vi "Read OPC UA Client Refnum.vi"(8 "error in (no error)":errorcluster, 11 "UA Server in":refnum<class "UA Server.lvclass">) -> (0 "error out":errorcluster, 2 "OPC UA client refnum":T1, 3 "UA Server out":refnum<class "UA Server.lvclass">)   [LabVIEW 2017, in "Browser Core.lvlib" / "UA Server.lvclass"]
uses:
  UA Server.lvclass
  <vilib>/OPCUA/controls/OPC UA Client Refnum.ctl
  UA Server.lvclass/UA Server.ctl
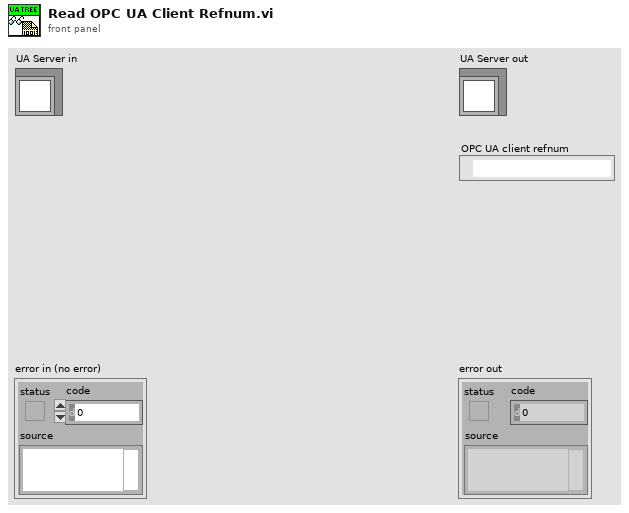
[diagram p1: front panel]
types:
  T1 = typedef "OPC UA Client Refnum.ctl" = refnum<k21>
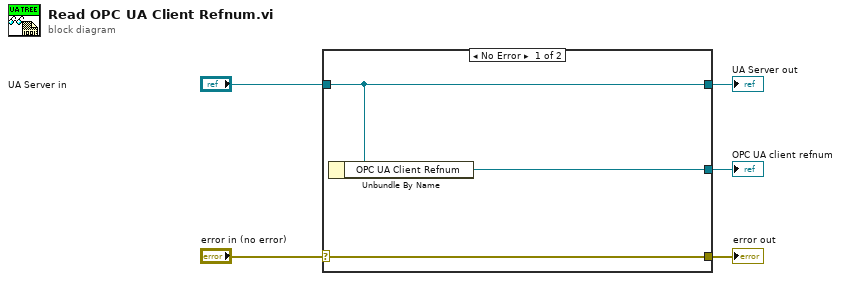
[diagram p0: block diagram]
diagram:
  n1 = case shown="No Error" "error in (no error)" {
    selector: "error in (no error)" -> [w8 w9]
    tunnel: [w8 w9] -> w4
    tunnel: [w7 w10] -> w2
    tunnel: "UA Server in" -> [w7 w10]
    tunnel: [w6 _] -> w1
    frame No Error {
      n2 = Unbundle By Name(w7) -> ("OPC UA Client Refnum"=w6:T1)
    }
    frame Error {
    }
  }
  "error out" <- w4
  "UA Server out" <- w2
  "OPC UA client refnum" <- w1
